vi "FdxLoginCvi.vi"(4 "ClApplicationVersion":string, 5 "Privileges":u32(ring)=4294967295 items=["PRIVILEGES_ADMIN"=4294967295], 6 "ClApplication":string, 7 "ClUser":string, 8 "error in":errorcluster, 9 "ClHostName":string, 10 "SrvName":string, 11 "ResourceID":u32) -> (0 "error out":errorcluster, 3 "InstrumentHandle":u32)   [LabVIEW 2020, in "AIM664LV.lvlib"]
doc: "This function provides log in to a resource."
uses:
  AIM664LV.lvlib
  FdxGlobalDllPath.vi
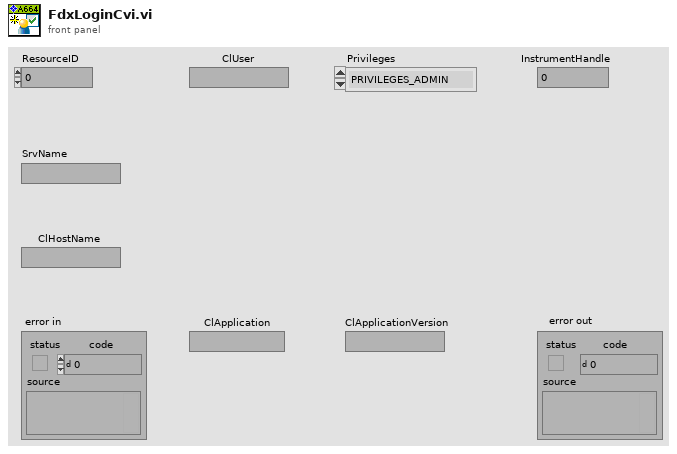
[diagram p1: front panel]
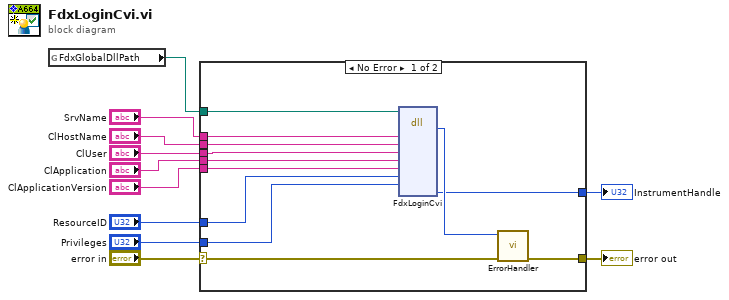
[diagram p0: block diagram]
diagram:
  n1 = global read "FdxGlobalDllPath.vi" "FdxGlobalDllPath"() -> (w9:path)
  n2 = case shown="No Error" "error in" {
    selector: "error in" -> [w22 w24]
    tunnel: [w23 w24] -> w11
    tunnel: w9 -> [w20 _]
    tunnel: [w19 _] -> w8
    tunnel: "SrvName" -> [w18 _]
    tunnel: "ClHostName" -> [w17 _]
    tunnel: "ClUser" -> [w16 _]
    tunnel: "ClApplication" -> [w15 _]
    tunnel: "ClApplicationVersion" -> [w14 _]
    tunnel: "ResourceID" -> [w13 _]
    tunnel: "Privileges" -> [w12 _]
    frame No Error {
      n3 = dll-call lib="aim_fdx.19.dll" fn="FdxLoginCvi"(path in=w20, "SrvName"=w18, "ClHostName"=w17, "ClUser"=w16, "ClApplication"=w15, "ClApplicationVersion"=w14, "ResourceID"=w13, "Privileges"=w12) -> ("status"=w21:i32, "Handle"=w19:u32)  [unwired: 4 in, 8 out]
      n4 = call "ErrorHandler.vi"("error in"=w22, "AIM Error"=w21) -> ("error out"=w23:errorcluster)  [unwired: 9 in]
    }
    frame Error {
    }
  }
  "error out" <- w11
  "InstrumentHandle" <- w8
